vi "Szimulacio.vi"() -> ()   [LabVIEW 2013]
uses:
  Parameterek.ctl
panel:
  in  "mód":enum16{"szinusz", "ugrás"}(ring)=enum."ugrás"
  out "Hõáram a belsõ rétegen belül":dbl[][](graph)
  out "Hõáram a középsõ rétegen belül":dbl[][](graph)
  out "F bel_in":dbl[](graph) caption="Hõáram a a belsõ falon befelé"
  out "F kozbel":dbl[](graph) caption="Hõáram a középsõ és belsõ réteg között"
  out "F kulkoz":dbl[](graph) caption="Hõáram a külsõ és középsõ réteg között"
  out "Hõáram a külsõ PCM rétegen belül":dbl[][](graph)
  out "Hõáram  a falon befelé":dbl[](graph)
  in  "t_sim [nap]":dbl=14.0
  out "Q_belsolevego":dbl[](graph) caption="Belsõ levegõ hõtartalma"
  out "T_belsolevego":dbl[](graph) caption="Belsõ levegõ hõmérséklete"
  out "T_belso":dbl[][](graph) caption="Belsõ PCM rétegek hõmérséklete"
  out "Q_belso":dbl[][](graph) caption="Belsõ PCM rétegek hõtartalma"
  out "T_kulso":dbl[][](graph) caption="Külsõ PCM rétegek hõmérséklete"
  out "Q_kulso":dbl[][](graph) caption="Külsõ PCM rétegek hõtartalma"
  in  "Parameterek":T1={"rholevego"=0.0, "Vlevego"=0.0, "Mlevego"=0.0, "clevego"=0.0, "rho PCM"=1100.0, "rho kulso"=28.3, "Dkulso"=0.1, "nkulso"=10, "dkulso"=0.0, "vkulso"=0.0, "rho kozepso"=28.3, "Dkozepso"=0.06, "nkozepso"=6, "dkozepso"=0.0, "vkozepso"=0.0, "mkozepso"=0.0, "mkulso"=0.0, "rho belso"=28.3, "Dbelso"=0.1, "nbelso"=10, "dbelso"=0.0, "vbelso"=0.0, "mbelso"=0.0, "Xpcm_kulso"=0.3, "Xpcm_belso"=0.3, "mpcm_kulso"=0.0, "mpcm_belso"=0.0, "mkulso_pcm"=0.0, "mbelso_pcm"=0.0, "ckulso"=1.13, "ckozepso"=1.13, "cbelso"=1.13, "cpcm_szilard"=1.9, "cpcm_foly"=1.5, "ckulso_Topalatt"=0.0, "cbelso_Topalatt"=0.0, "ckulso_Topfelett"=0.0, "cbelso_Topfelett"=0.0, "hpcm_olv"=140.0, "ckulso_eff_Tolv"=0.0, "cbelso_eff_Tolv"=0.0, "Qkulso_op_also"=0.0, "Qkulso_op_felso"=0.0, "Qbelso_op_also"=0.0, "Qbelso_op_felso"=0.0, "lambda_kulso"=5e-05, "lambda_kozepso"=5e-05, "lambda_belso"=5e-05, "lambda_pcm"=0.00018, "VXpcm_kulso"=0.0, "VXpcm_belso"=0.0, "lambda_kulsoPCM"=0.0, "lambda_belsoPCM"=0.0, "Alfa_kulso"=0.015, "Alfa_belso"=0.006, "Alfa_kont"=0.03, "Top_also"=24.0, "Top_felso"=28.0, "cpcm_olvnelkul"=0.0, "Tbelsolevego_0"=22.0}
  out "T_kozepso":dbl[][](graph) caption="Középsõ rétegek hõmérséklete"
  out "T_kulsolevego":dbl[](graph)
  out "Q_kozepso":dbl[][](graph) caption="Középsõ rétegek hõtartalma"
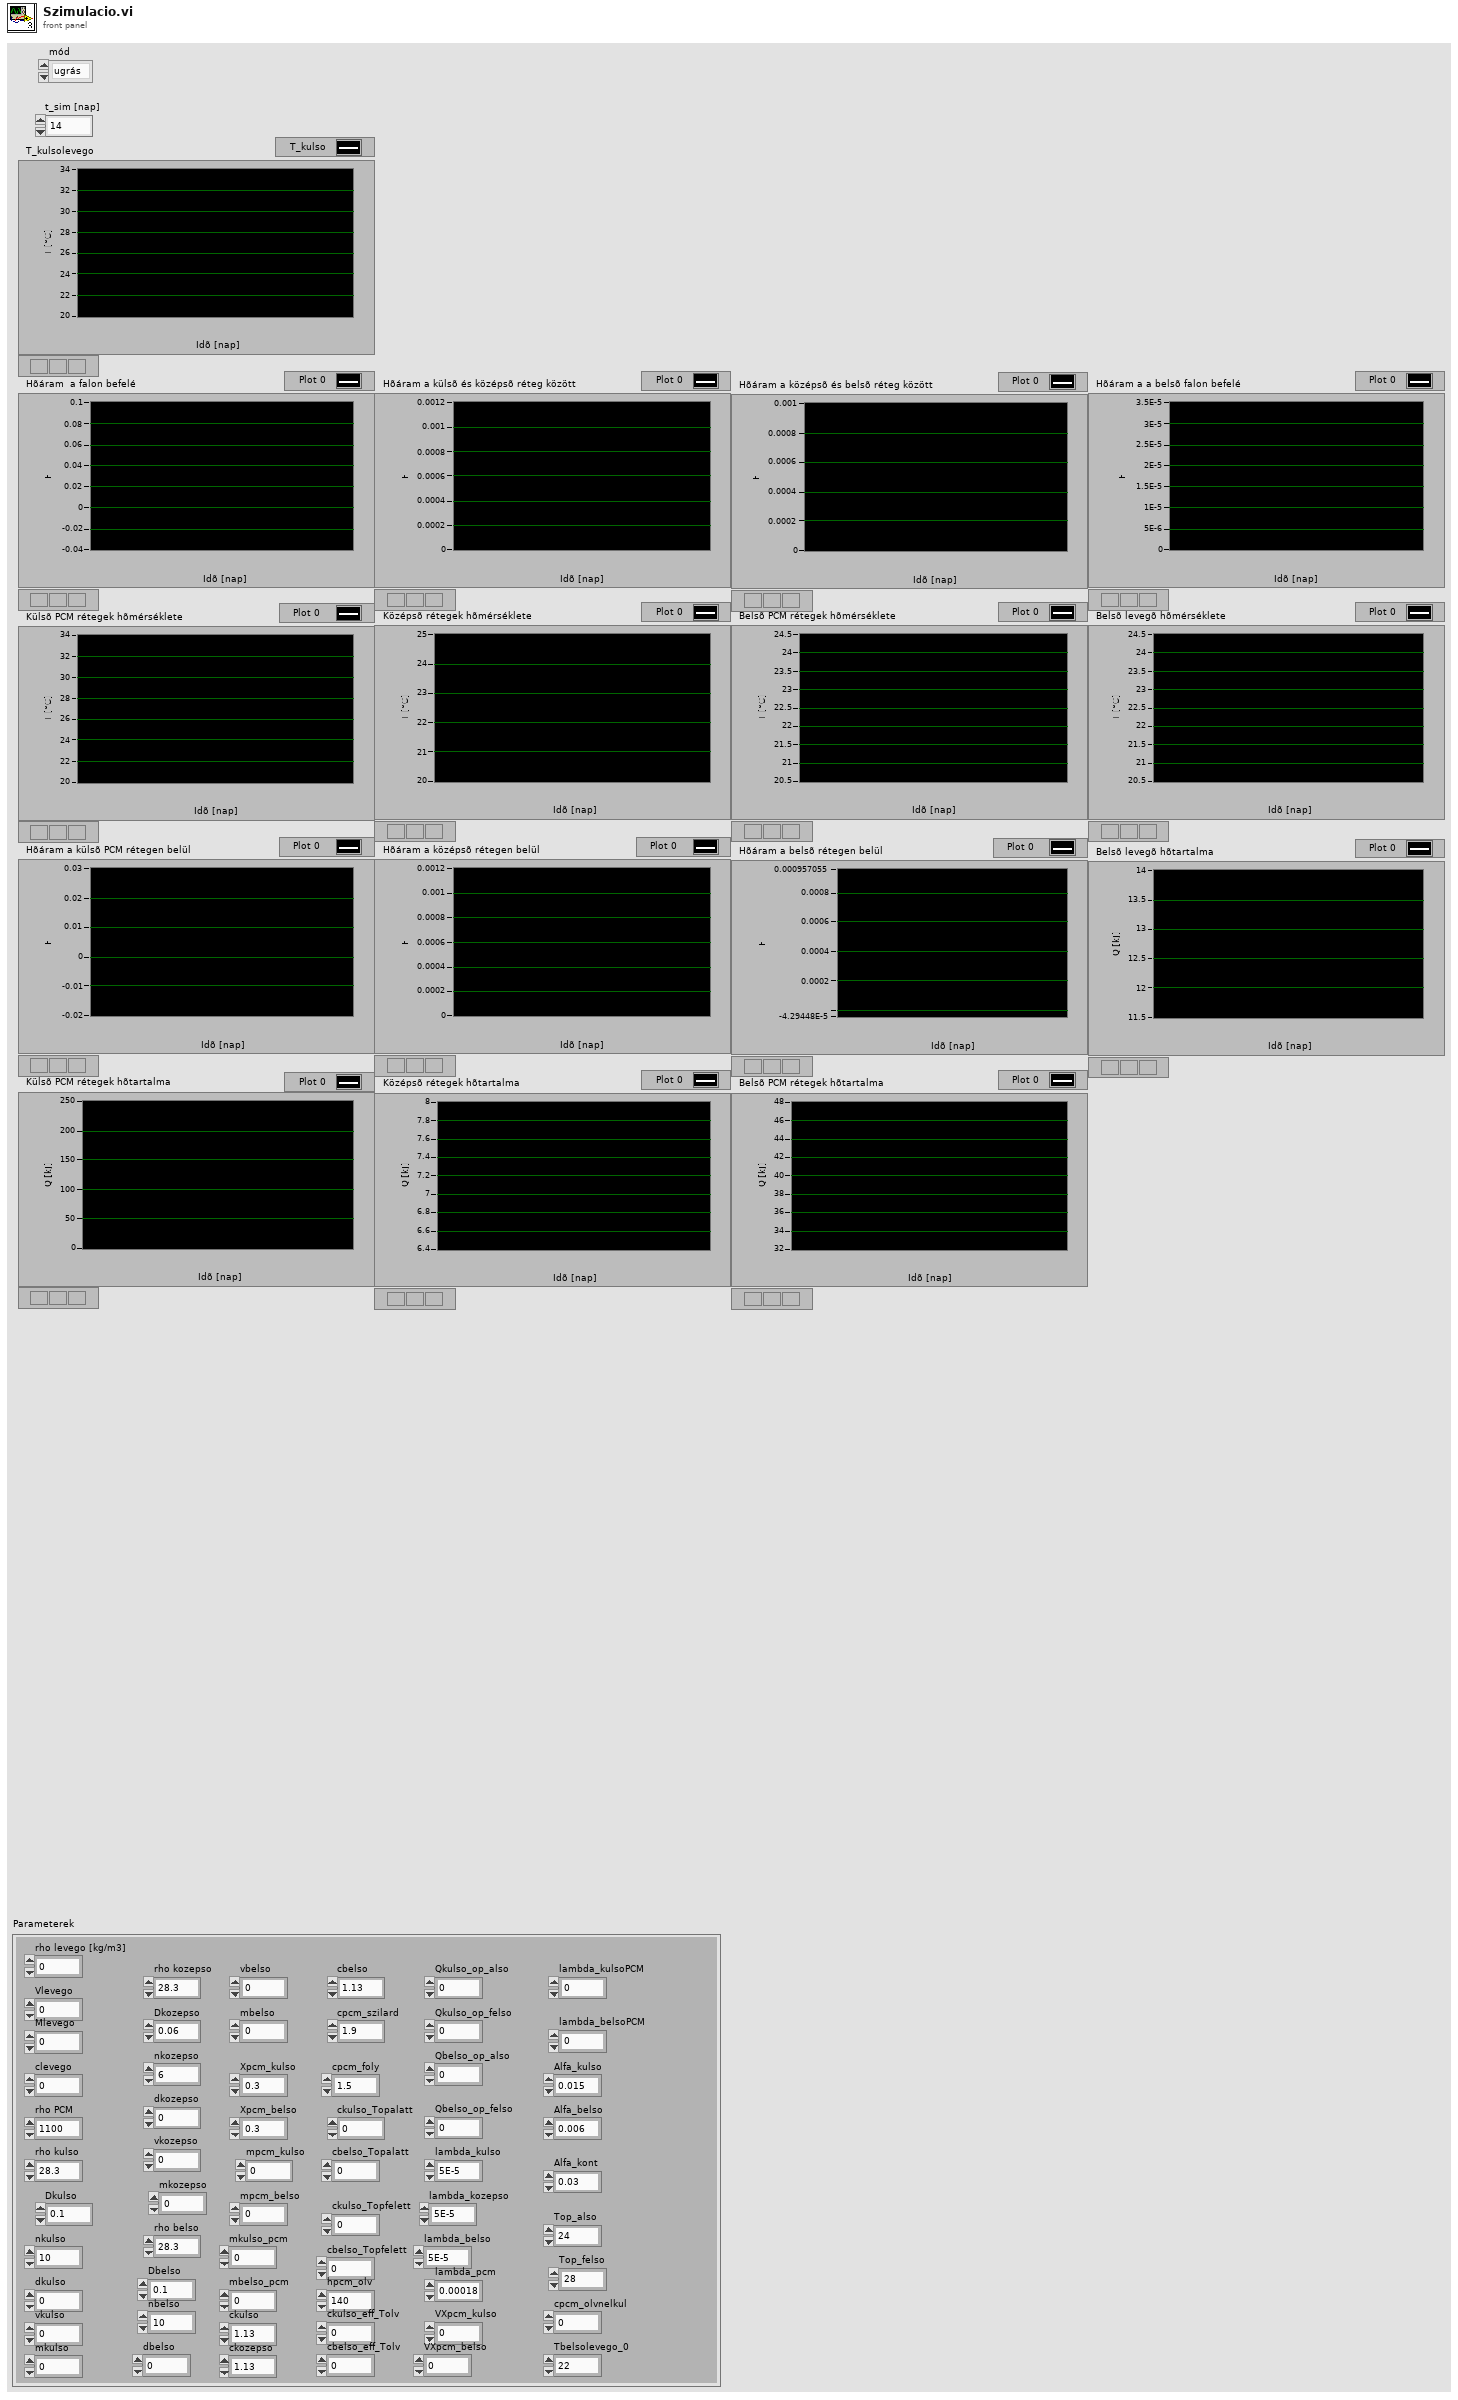
[diagram p1: front panel]
types:
  T1 = typedef "Parameterek.ctl" = cluster{"rholevego":dbl, "Vlevego":dbl, "Mlevego":dbl, "clevego":dbl, "rho PCM":dbl, "rho kulso":dbl, "Dkulso":dbl, "nkulso":i32, "dkulso":dbl, "vkulso":dbl, "rho kozepso":dbl, "Dkozepso":dbl, "nkozepso":i32, "dkozepso":dbl, "vkozepso":dbl, "mkozepso":dbl, "mkulso":dbl, "rho belso":dbl, "Dbelso":dbl, "nbelso":i32, "dbelso":dbl, "vbelso":dbl, "mbelso":dbl, "Xpcm_kulso":dbl, "Xpcm_belso":dbl, "mpcm_kulso":dbl, "mpcm_belso":dbl, "mkulso_pcm":dbl, "mbelso_pcm":dbl, "ckulso":dbl, "ckozepso":dbl, "cbelso":dbl, "cpcm_szilard":dbl, "cpcm_foly":dbl, "ckulso_Topalatt":dbl, "cbelso_Topalatt":dbl, "ckulso_Topfelett":dbl, "cbelso_Topfelett":dbl, "hpcm_olv":dbl, "ckulso_eff_Tolv":dbl, "cbelso_eff_Tolv":dbl, "Qkulso_op_also":dbl, "Qkulso_op_felso":dbl, "Qbelso_op_also":dbl, "Qbelso_op_felso":dbl, "lambda_kulso":dbl, "lambda_kozepso":dbl, "lambda_belso":dbl, "lambda_pcm":dbl, "VXpcm_kulso":dbl, "VXpcm_belso":dbl, "lambda_kulsoPCM":dbl, "lambda_belsoPCM":dbl, "Alfa_kulso":dbl, "Alfa_belso":dbl, "Alfa_kont":dbl, "Top_also":dbl, "Top_felso":dbl, "cpcm_olvnelkul":dbl, "Tbelsolevego_0":dbl}
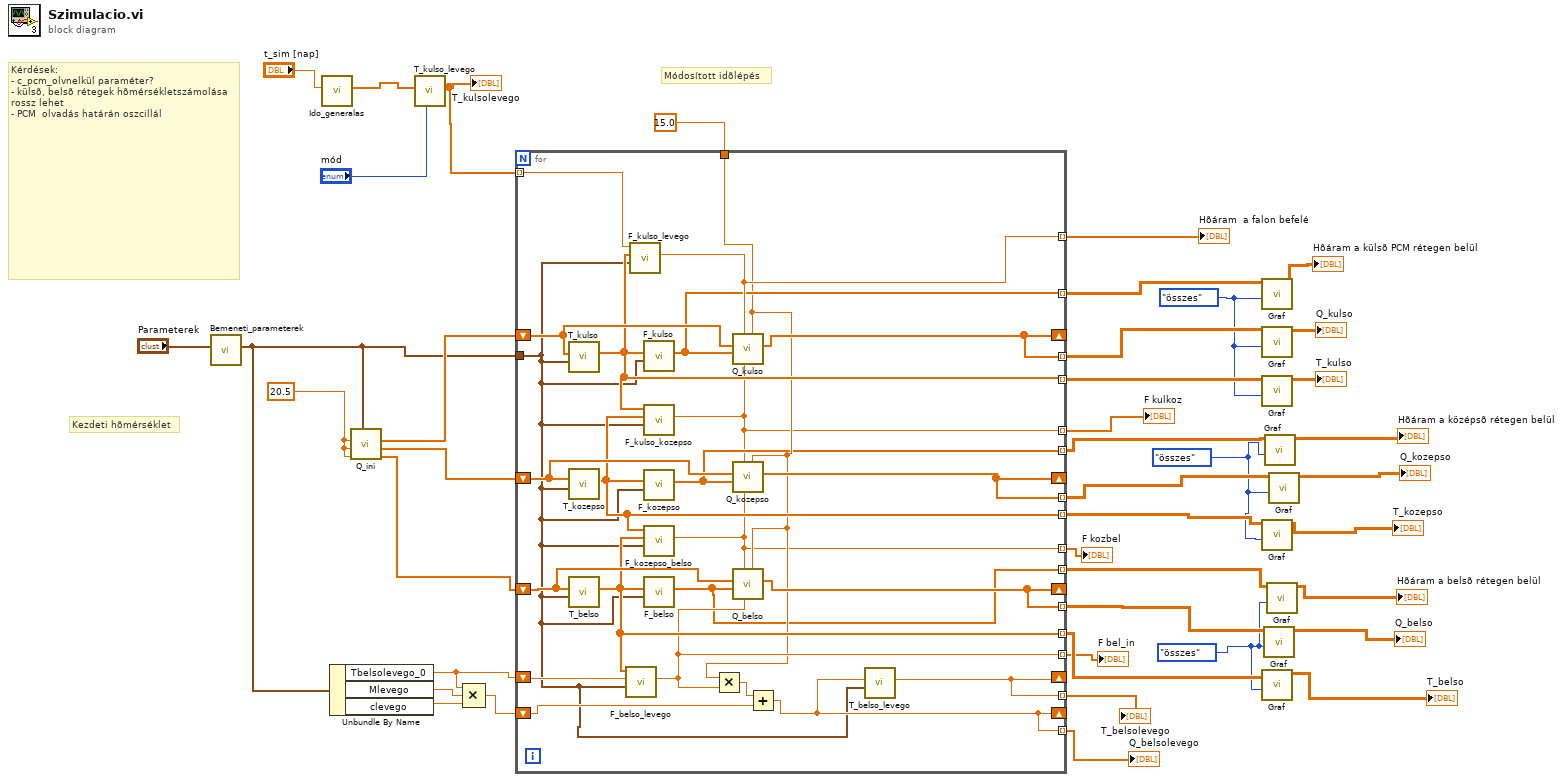
[diagram p0: block diagram]
diagram:
  w3 = enum16{"három", "összes", "eleje", "vége"}."összes" ("mód")
  w7 = enum16{"három", "összes", "eleje", "vége"}."összes" ("mód")
  w19 = enum16{"három", "összes", "eleje", "vége"}."összes" ("mód")
  w41 = 20.5 ("Q_kulso_0")
  # "Módosított idõlépés"
  # "Kérdések: \n- c_pcm_olvnelkül paraméter?\n- külsõ, belsõ rétegek hõmérsékletszámolása rossz lehet\n- PCM  olvadás határán oszcillál"
  # "Kezdeti hõmérséklet"
  n1 = call "Bemeneti_parameterek.vi"("Parameterek"="Parameterek") -> ("Parameterek 2"=w33:T1)  [unwired: 10 in]
  n2 = call "Ido_generalas.vi"("t_sim [nap]"="t_sim [nap]") -> ("t_vektor"=w27:dbl[])  [unwired: 10 in]
  n3 = Unbundle By Name(w33) -> ("Tbelsolevego_0"=w34:dbl, "Mlevego"=w32:dbl, "clevego"=w31:dbl)
  n4 = call "Q_ini.vi"("Parameterek"=w33, "T_belso_0"=w41, "T_kozepso_0"=w41, "T_kulso_0"=w41) -> ("Q_belso_0_vektor"=w38:dbl[], "Q_kozepso_0_vektor"=w39:dbl[], "Q_kulso_0 vektor"=w40:dbl[])  [unwired: 5 in]
  n5 = call "T_kulso_levego.vi"("mód"="mód", "t_vektor"=w27) -> ("T_kulso_levego_vektor"=w24:dbl[])  [unwired: 8 in, 1 out]
  "T_kulsolevego" <- w24
  n6 = Compound Arithmetic op=MULTIPLY(w34, w32, w31) -> (w35:dbl)
  n7 = for {
    tunnel: w24 -> [w65] mode=indexing
    shift-right: [w64] -> _
    shift-left: w39 -> [w66]
    tunnel: [w64] -> w17 mode=indexing
    tunnel: [w58] -> w16 mode=indexing
    tunnel: w33 -> [w48]
    shift-right: [w62] -> _
    shift-left: w40 -> [w63]
    shift-right: [w60] -> _
    shift-left: w38 -> [w61]
    tunnel: [w62] -> w21 mode=indexing
    tunnel: [w59] -> w20 mode=indexing
    tunnel: [w60] -> w14 mode=indexing
    tunnel: [w57] -> w12 mode=indexing
    shift-right: [w53] -> _
    shift-left: w34 -> [w56]
    shift-right: [w52] -> _
    shift-left: w35 -> [w55]
    tunnel: [w53] -> w36 mode=indexing
    tunnel: [w52] -> w30 mode=indexing
    tunnel: [w51] -> w29 mode=indexing
    tunnel: [w50] -> w28 mode=indexing
    tunnel: [w44] -> w26 mode=indexing
    tunnel: [w43] -> w10 mode=indexing
    tunnel: [w49] -> w9 mode=indexing
    tunnel: 15.0 ("dt") -> [w47]
    tunnel: [w46] -> w6 mode=indexing
    tunnel: [w45] -> w2 mode=indexing
    n8 = call "T_kulso.vi"("Parameterek"=w48, "Q kulso vektor"=w63) -> ("T kulso vektor"=w59:dbl[])  [unwired: 9 in]
    n9 = call "T_kozepso.vi"("Parameterek"=w48, "Q kozepso vektor"=w66) -> ("T kozepso vektor"=w58:dbl[])  [unwired: 9 in]
    n10 = call "T_belso.vi"("Parameterek"=w48, "Q belso vektor"=w61) -> ("T belso vektor"=w57:dbl[])  [unwired: 9 in]
    n11 = call "F_belso_levego.vi"("Parameterek"=w48, "T_belso_levego"=w56, "T_belso_vektor"=w57) -> ("F_fal_belso_levego"=w49:dbl)  [unwired: 8 in]
    n12 = call "F_kulso_levego.vi"("Parameterek"=w48, "T_kulso_vektor"=w59, "T_kulso_levego"=w65) -> ("F_kulso_levego_fal"=w51:dbl)  [unwired: 8 in]
    n13 = call "F_kulso.vi"("Parameterek"=w48, "T_kulso_vektor"=w59) -> ("F_kulso_vektor"=w50:dbl[])  [unwired: 9 in]
    n14 = call "F_kulso_kozepso.vi"("T_kulso_vektor"=w59, "T_kozepso_vektor"=w58, "Parameterek"=w48) -> ("F_10_11"=w44:dbl)  [unwired: 7 in]
    n15 = call "F_kozepso.vi"("Parameterek"=w48, "T_kozepso_vektor"=w58) -> ("F_kozepso_vektor"=w46:dbl[])  [unwired: 9 in]
    n16 = call "F_kozepso_belso.vi"("T_kozepso_vektor"=w58, "T_belso_vektor"=w57, "Parameterek"=w48) -> ("F_16_17"=w43:dbl)  [unwired: 7 in]
    n17 = call "F_belso.vi"("Parameterek"=w48, "T_belso_vektor"=w57) -> ("F_belso_vektor"=w45:dbl[])  [unwired: 9 in]
    n18 = Multiply(x=w47, y=w49) -> (x*y=w54:dbl)
    n19 = call "Q_kulso.vi"("idolepes"=w47, "F_10_11"=w44, "F_kulso_levego_fal"=w51, "F_kulso_vektor"=w50, "Q_kulso_elozo_vektor"=w63) -> ("Q_kulso_aktualis_vektor"=w62:dbl[])  [unwired: 6 in]
    n20 = call "Q_kozepso.vi"("idolepes"=w47, "F_kozbel"=w43, "F_kulkoz"=w44, "F_kozepso_vektor"=w46, "Q_kozepso_elozo_vektor"=w66) -> ("Q_kozepso_aktualis_vektor"=w64:dbl[])  [unwired: 6 in]
    n21 = call "Q_belso.vi"("idolepes"=w47, "F_belso_fal"=w49, "F_16_17"=w43, "F_belso_vektor"=w45, "Q_belso_elozo_vektor"=w61) -> ("Q_belso_aktualis_vektor"=w60:dbl[])  [unwired: 6 in]
    n22 = Add(x=w54, y=w55) -> (x+y=w52:dbl)
    n23 = call "T_belso_levego.vi"("Parameterek"=w48, "Q_belsolevego"=w52) -> ("T_belsolevego"=w53:dbl)  [unwired: 9 in]
  }
  "T_belsolevego" <- w36
  "Q_belsolevego" <- w30
  "Hõáram  a falon befelé" <- w29
  "F kulkoz" <- w26
  "F kozbel" <- w10
  "F bel_in" <- w9
  n24 = call "Graf.vi"("mód"=w19, "F_kulso_vektor"=w28) -> ("Grafikonra"=→"Hõáram a külsõ PCM rétegen belül":dbl[][])  [unwired: 9 in]
  n25 = call "Graf.vi"("mód"=w19, "F_kulso_vektor"=w21) -> ("Grafikonra"=→"Q_kulso":dbl[][])  [unwired: 9 in]
  n26 = call "Graf.vi"("mód"=w19, "F_kulso_vektor"=w20) -> ("Grafikonra"=→"T_kulso":dbl[][])  [unwired: 9 in]
  n27 = call "Graf.vi"("mód"=w7, "F_kulso_vektor"=w16) -> ("Grafikonra"=→"T_kozepso":dbl[][])  [unwired: 9 in]
  n28 = call "Graf.vi"("mód"=w3, "F_kulso_vektor"=w12) -> ("Grafikonra"=→"T_belso":dbl[][])  [unwired: 9 in]
  n29 = call "Graf.vi"("mód"=w3, "F_kulso_vektor"=w14) -> ("Grafikonra"=→"Q_belso":dbl[][])  [unwired: 9 in]
  n30 = call "Graf.vi"("mód"=w7, "F_kulso_vektor"=w6) -> ("Grafikonra"=→"Hõáram a középsõ rétegen belül":dbl[][])  [unwired: 9 in]
  n31 = call "Graf.vi"("mód"=w3, "F_kulso_vektor"=w2) -> ("Grafikonra"=→"Hõáram a belsõ rétegen belül":dbl[][])  [unwired: 9 in]
  n32 = call "Graf.vi"("mód"=w7, "F_kulso_vektor"=w17) -> ("Grafikonra"=→"Q_kozepso":dbl[][])  [unwired: 9 in]
